vi "Get Fixed & Fitted Parameters.vi"(8 "Error In":errorcluster, 11 "All Parameter Constraints":T4) -> (0 "Error Out":errorcluster, 3 "All Parameter Constraints with Values":T1)   [LabVIEW 2021, in "Fits.lvlib"]
uses:
  Fits.lvlib
  IRF(X)PSED/Decay Fit Parameter Constraints Arrays.ctl
  IRF(X)PSED/Decay Fit Parameters In List.ctl
  Decay Model.ctl
  IRF(X)PSED/Decay Fit Parameter Constraints with Values.ctl
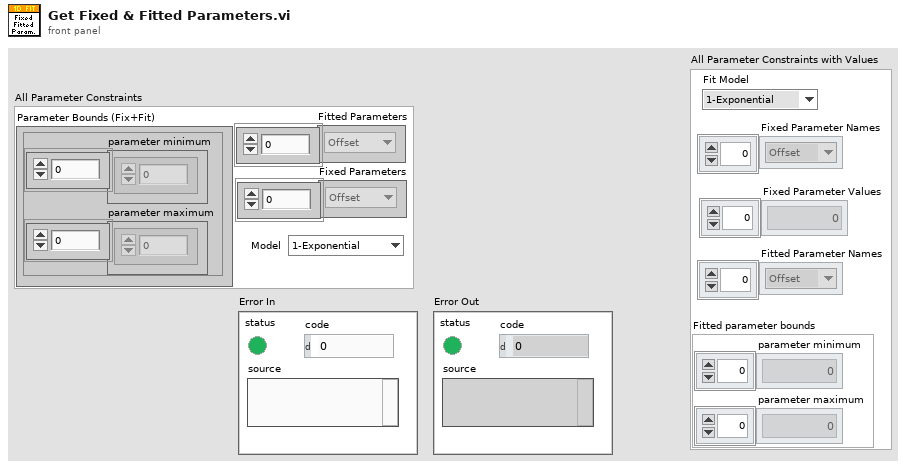
[diagram p1: front panel]
types:
  T1 = typedef "Fits.lvlib/Decay Fit Parameter Constraints with Values.ctl" = cluster{"Fitted parameter bounds":cluster{"parameter minimum":dbl[], "parameter maximum":dbl[]}, "Fixed Parameter Values":dbl[], "Fixed Parameter Names":T2[], "Fitted Parameter Names":T2[], "Fit Model":T3}
  T2 = typedef "Fits.lvlib/Decay Fit Parameters In List.ctl" = enum16{"Offset", "Baseline", "A_1", "tau_1", "A_2", "tau_2"}
  T3 = typedef "Fits.lvlib/Decay Model.ctl" = enum16{"1-Exponential", "2-Exponentials"}
  T4 = typedef "Fits.lvlib/Decay Fit Parameter Constraints Arrays.ctl" = cluster{"Parameter Bounds (Fix+Fit)":cluster{"parameter minimum":dbl[], "parameter maximum":dbl[]}, "Fitted Parameters":T2[], "Fixed Parameters":T2[], "Fit Model":T3}
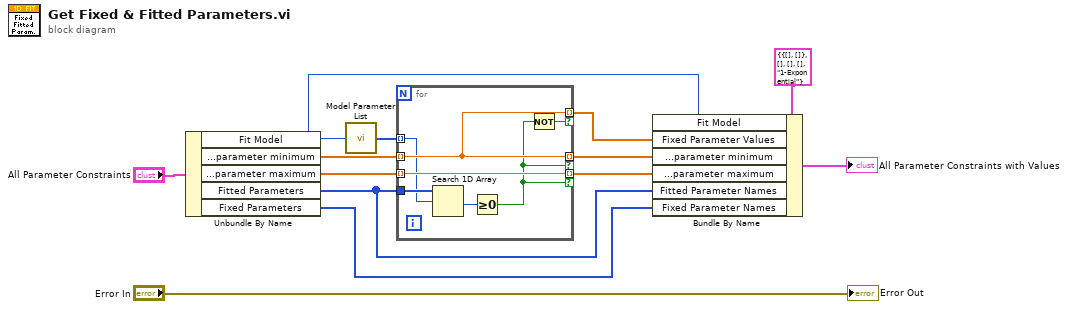
[diagram p0: block diagram]
diagram:
  n1 = Unbundle By Name("All Parameter Constraints") -> ("Fit Model"=w9:T3, "Parameter Bounds (Fix+Fit).parameter minimum"=w12:dbl[], "Parameter Bounds (Fix+Fit).parameter maximum"=w11:dbl[], "Fitted Parameters"=w5:T2[], "Fixed Parameters"=w4:T2[])
  n2 = call "Model Parameter List.vi"("Fit Model"=w9) -> ("Model Parameter List"=w10:T2[])
  n3 = for {
    tunnel: w12 -> [w17] mode=indexing
    tunnel: w11 -> [w18] mode=indexing
    tunnel: w10 -> [w16] mode=indexing
    tunnel: w5 -> [w20]
    tunnel: [w17] -> w7 mode=indexing if=w15
    tunnel: [w18] -> w6 mode=indexing if=w15
    tunnel: [w17] -> w8 mode=indexing if=w14
    n4 = Search 1D Array(1D array=w20, element=w16) -> (index of element=w19:i32)  [unwired: 1 in]
    n5 = Greater Or Equal To 0?(x=w19) -> (x >= 0?=w15:bool)
    n6 = Not(x=w15) -> (.not. x?=w14:bool)
  }
  n7 = Bundle By Name(cluster=T1 {"Fitted parameter bounds"={"parameter minimum"=[], "parameter maximum"=[]}, "Fixed Parameter Values"=[], "Fixed Parameter Names"=[], "Fitted Parameter Names"=[], "Fit Model"=enum."1-Exponential"} ("All Parameter Constraints with Values"), "Fit Model"=w9, "Fixed Parameter Values"=w8, "Fitted parameter bounds.parameter minimum"=w7, "Fitted parameter bounds.parameter maximum"=w6, "Fitted Parameter Names"=w5, "Fixed Parameter Names"=w4) -> (→"All Parameter Constraints with Values":T1)
  "Error Out" <- "Error In"
